vi "Write HulkNumber.vi"(8 "error in (no error)":errorcluster, 10 "HulkNumber":dbl, 11 "Hulk Hogan in":refnum<class "Hulk Hogan.lvclass">) -> (0 "error out":errorcluster, 3 "Hulk Hogan out":refnum<class "Hulk Hogan.lvclass">)   [LabVIEW 2019, in "Hulk Hogan.lvclass"]
uses:
  Hulk Hogan.lvclass
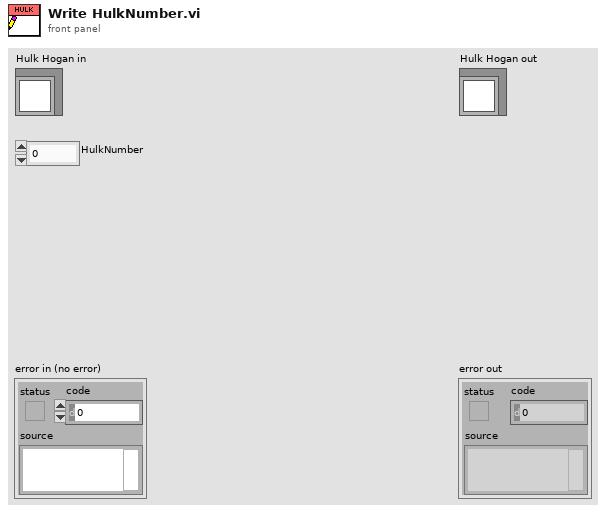
[diagram p1: front panel]
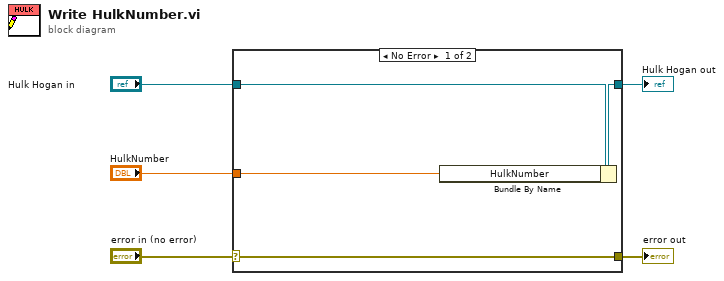
[diagram p0: block diagram]
diagram:
  n1 = case shown="No Error" "error in (no error)" {
    selector: "error in (no error)" -> [w9 w10]
    tunnel: [w9 w10] -> w4
    tunnel: [w7 w11] -> w2
    tunnel: "Hulk Hogan in" -> [w8 w11]
    tunnel: "HulkNumber" -> [w6 _]
    frame No Error {
      n2 = Bundle By Name(cluster=w8, "HulkNumber"=w6) -> (w7:refnum<class "Hulk Hogan.lvclass">)
    }
    frame Error {
    }
  }
  "error out" <- w4
  "Hulk Hogan out" <- w2
